vi "Low-Level Read.vi"(8 "error in (no error)":errorcluster, 9 "timeout ms (5000)":i32=5000, 11 "WebSockets in":refnum<class "WebSocket.lvclass">) -> (0 "error out":errorcluster, 1 "Opcode":T1=1 items=["Cont. Frame"=0, "Text"=1, "Binary"=2, "Ping"=9, "Pong"=10], 2 "Data":string, 3 "WebSockets out":refnum<class "WebSocket.lvclass">, 4 "Finished?":bool)   [LabVIEW 2013, in "WebSockets.lvlib" / "WebSocket.lvclass"]
doc: "Reads and decodes an incoming WebSockets message.\n\nOpcode: Opcode for the message.\nData: Contains the WebSockets payload\nFinished?: Determines whether the message is complete for fragmented messages. If false, must continue to read messages (continuation frames with opcode = 0) until Finished? is true."
uses:
  WebSocket.lvclass
  Opcodes.ctl
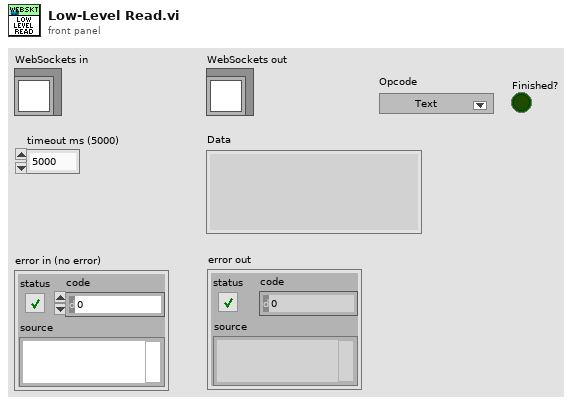
[diagram p1: front panel]
types:
  T1 = typedef "WebSockets.lvlib/WebSocket.lvclass/Opcodes.ctl" = u8
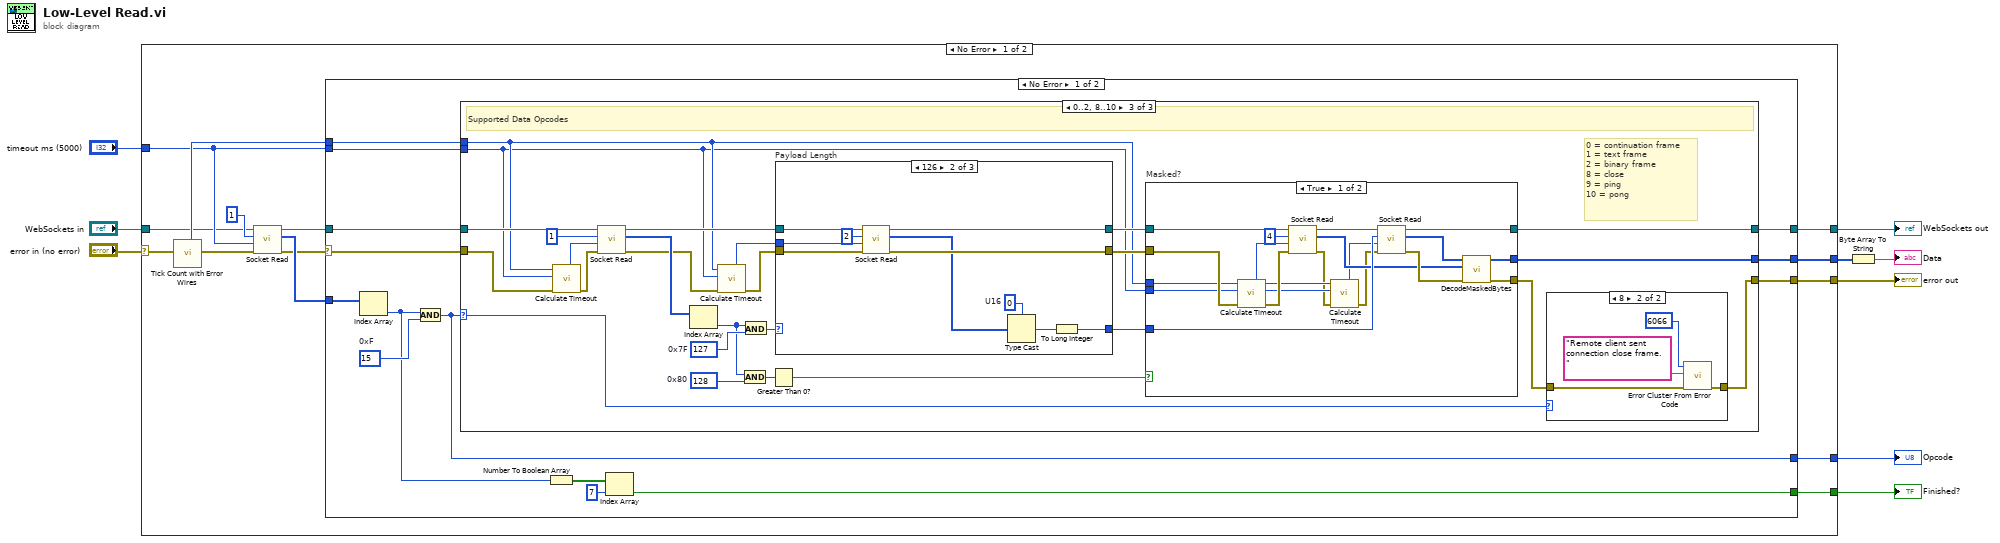
[diagram p0: block diagram]
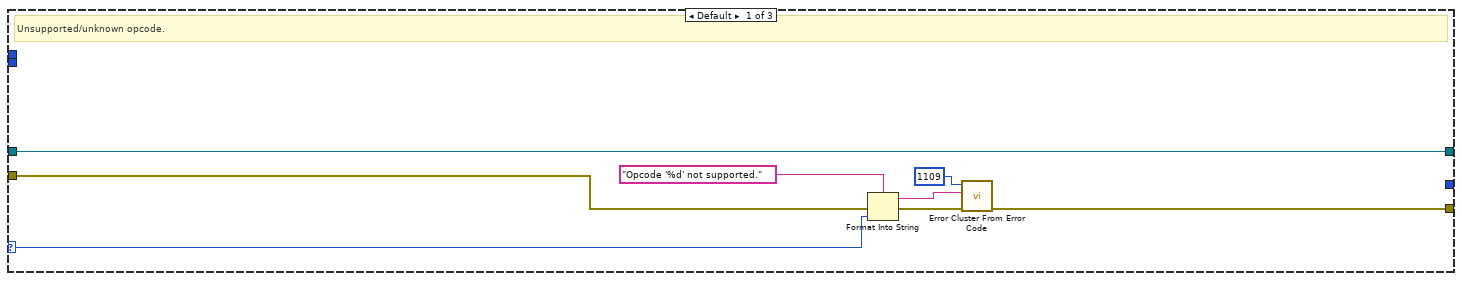
[diagram p2: hidden frame]
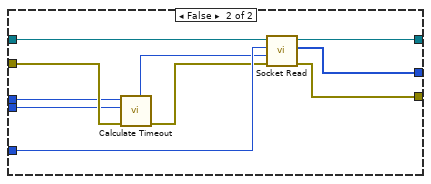
[diagram p5: hidden frame]
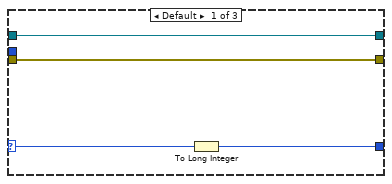
[diagram p6: hidden frame]
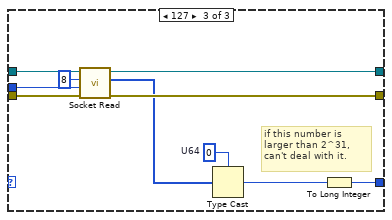
[diagram p7: hidden frame]
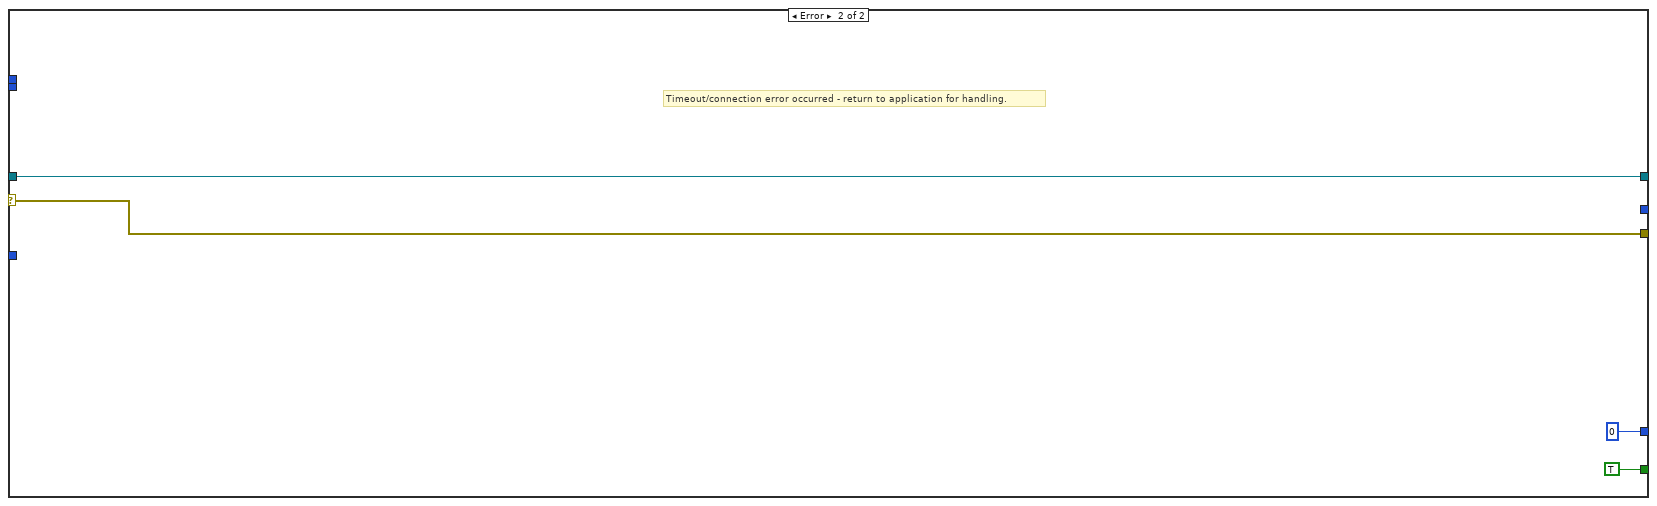
[diagram p8: hidden frame]
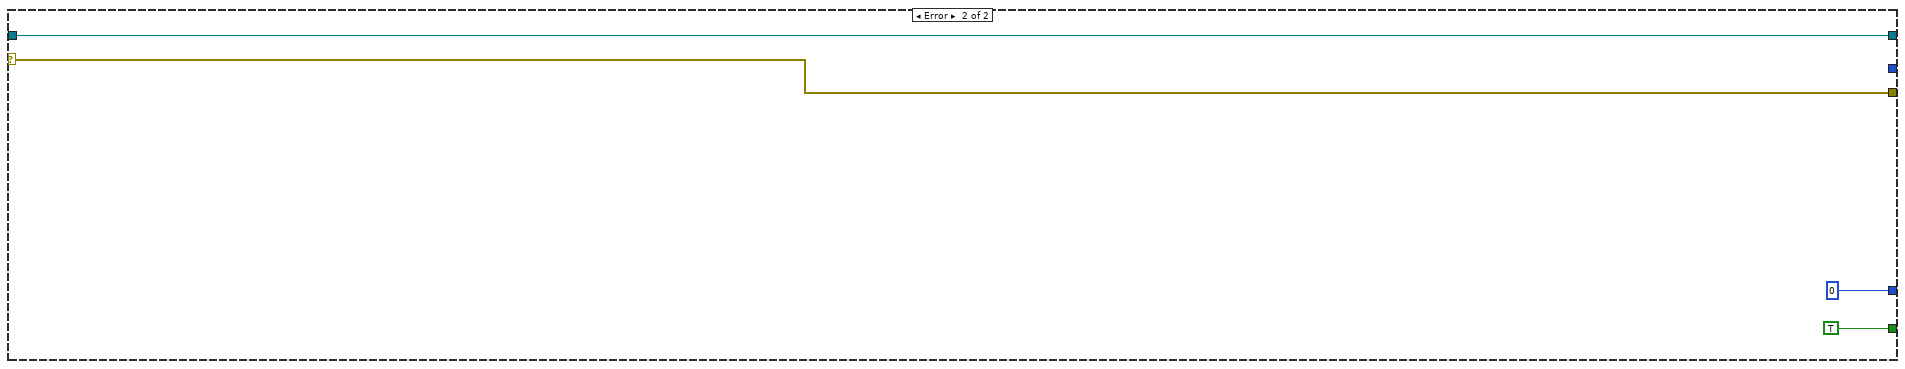
[diagram p9: hidden frame]
diagram:
  n1 = case shown="No Error" "error in (no error)" {
    selector: "error in (no error)" -> [w19 w138]
    tunnel: [w23 _] -> w9
    tunnel: [w22 w138] -> w7
    tunnel: "timeout ms (5000)" -> [w15 _]
    tunnel: [w21 u8 0] -> w4
    tunnel: [w20 TRUE] -> w5
    tunnel: "WebSockets in" -> [w11 w135]
    tunnel: [w10 w135] -> w1
    frame No Error {
      n2 = call "Tick Count with Error Wires.vi"("error in (no error)"=w19) -> ("error out"=w17:errorcluster, "millisecond timer value"=w18:u32)  [unwired: 9 in]
      n3 = call "Socket Read.vi"("error in (no error)"=w17, "timeout ms (5000)"=w15, "# bytes to read"=1 ("bytes to read"), "WebSocket in"=w11) -> ("error out"=w13:errorcluster, "Read Bytes"=w14:u8[], "WebSocket out"=w12:refnum<class "WebSocket.lvclass">)  [unwired: 5 in]
      n4 = case shown="No Error" w13 {
        selector: w13 -> [w33 w133]
        tunnel: w14 -> [w25 _]
        tunnel: w12 -> [w37 w134]
        tunnel: [w36 w134] -> w10
        tunnel: [w35 _] -> w23
        tunnel: [w34 w133] -> w22
        tunnel: [w31 u8 0] -> w21
        tunnel: [w28 TRUE] -> w20
        tunnel: w15 -> [w27 _]
        tunnel: w18 -> [w24 _]
        frame No Error {
          w32 = u8 15  # 0xF
          n5 = Index Array(array=w25) -> (element=w30:u8)  [unwired: 1 in]
          n6 = And(x=w30, y=w32) -> (x .and. y?=w31:u8)
          n7 = case shown="0..2, 8..10" w31 {
            selector: w31 -> [w39 _ w60]
            tunnel: w37 -> [w45 w46 w66]
            tunnel: [w45 w46 w73] -> w36
            tunnel: [_ _ w67] -> w35
            tunnel: [w44 w47 w58] -> w34
            tunnel: w33 -> [w43 w47 w55]
            tunnel: w27 -> [_ _ w48]
            tunnel: w24 -> [_ _ w49]
            frame Default {
              # "Unsupported/unknown opcode."
              n8 = Format Into String(format string="Opcode '%d' not supported.", error in=w43, w39) -> (resulting string=w41:string, error out=w42:errorcluster)  [unwired: 1 in]
              n9 = call <vilib>:"Error Cluster From Error Code.vi"("error in (no error)"=w42, "error message (\"\")"=w41, "error code (0)"=1109) -> ("error out"=w44:errorcluster)  [unwired: 6 in]
            }
            frame 3..7, 11..15 {
              # "3-7: Reserved non-control frames\n11-15: Reserved control frames"
              # "Reserved opcodes"
            }
            frame 0..2, 8..10 {
              w63 = u8 128  # 0x80
              w72 = u8 127  # 0x7F
              # "0 = continuation frame\n1 = text frame\n2 = binary frame\n8 = close\n9 = ping\n10 = pong"
              # "Supported Data Opcodes"
              n10 = call "Calculate Timeout.vi"("error in (no error)"=w55, "timeout ms"=w48, "t0"=w49) -> ("error out"=w54:errorcluster, "new timeout ms"=w52:i32)  [unwired: 6 in, 1 out]
              n11 = call "Socket Read.vi"("error in (no error)"=w54, "timeout ms (5000)"=w52, "# bytes to read"=1 ("bytes to read"), "WebSocket in"=w66) -> ("error out"=w53:errorcluster, "Read Bytes"=w57:u8[], "WebSocket out"=w65:refnum<class "WebSocket.lvclass">)  [unwired: 5 in]
              n12 = Index Array(array=w57) -> (element=w56:u8)  [unwired: 1 in]
              n13 = call "Calculate Timeout.vi"("error in (no error)"=w53, "timeout ms"=w48, "t0"=w49) -> ("error out"=w51:errorcluster, "new timeout ms"=w50:i32)  [unwired: 6 in, 1 out]
              n14 = And(x=w56, y=w63) -> (x .and. y?=w62:u8)
              n15 = And(x=w56, y=w72) -> (x .and. y?=w71:u8)
              n16 = Greater Than 0?(x=w62) -> (x > 0?=w61:bool)
              n17 = case "Payload Length" shown="126" w71 {
                selector: w71 -> [w109 _ _]
                tunnel: w65 -> [w110 w120 w129]
                tunnel: [w110 w119 w128] -> w70
                tunnel: [w108 w114 w127] -> w68
                tunnel: [w107 w117 w126] -> w69
                tunnel: w51 -> [w107 w116 w125]
                tunnel: w50 -> [_ w111 w121]
                frame Default {
                  n18 = To Long Integer(number=w109) -> (32bit integer=w108:i32)
                }
                frame 126 {
                  w113 = u16 0  # U16
                  n19 = call "Socket Read.vi"("error in (no error)"=w116, "timeout ms (5000)"=w111, "# bytes to read"=2 ("bytes to read"), "WebSocket in"=w120) -> ("error out"=w117:errorcluster, "Read Bytes"=w115:u8[], "WebSocket out"=w119:refnum<class "WebSocket.lvclass">)  [unwired: 5 in]
                  n20 = Type Cast(type=w113, x=w115) -> (*(type *) &x=w112:u16)
                  n21 = To Long Integer(number=w112) -> (32bit integer=w114:i32)
                }
                frame 127 {
                  w124 = u64 0  # U64
                  # "if this number is larger than 2^31, can't deal with it."
                  n22 = call "Socket Read.vi"("error in (no error)"=w125, "timeout ms (5000)"=w121, "# bytes to read"=8 ("bytes to read"), "WebSocket in"=w129) -> ("error out"=w126:errorcluster, "Read Bytes"=w122:u8[], "WebSocket out"=w128:refnum<class "WebSocket.lvclass">)  [unwired: 5 in]
                  n23 = Type Cast(type=w124, x=w122) -> (*(type *) &x=w123:u64)
                  n24 = To Long Integer(number=w123) -> (32bit integer=w127:i32)
                }
              }
              n25 = case "Masked?" shown="True" w61 {
                tunnel: [w96 w106] -> w73
                tunnel: w70 -> [w95 w105]
                tunnel: w69 -> [w86 w101]
                tunnel: w68 -> [w92 w104]
                tunnel: [w90 w102] -> w67
                tunnel: [w88 w103] -> w59
                tunnel: w49 -> [w83 w98]
                tunnel: w48 -> [w82 w97]
                frame True {
                  n26 = call "Calculate Timeout.vi"("error in (no error)"=w86, "timeout ms"=w82, "t0"=w83) -> ("error out"=w85:errorcluster, "new timeout ms"=w84:i32)  [unwired: 6 in, 1 out]
                  n27 = call "Socket Read.vi"("error in (no error)"=w85, "timeout ms (5000)"=w84, "# bytes to read"=4 ("bytes to read"), "WebSocket in"=w95) -> ("error out"=w81:errorcluster, "Read Bytes"=w87:u8[], "WebSocket out"=w94:refnum<class "WebSocket.lvclass">)  [unwired: 5 in]
                  n28 = call "Calculate Timeout.vi"("error in (no error)"=w81, "timeout ms"=w82, "t0"=w83) -> ("error out"=w80:errorcluster, "new timeout ms"=w79:i32)  [unwired: 6 in, 1 out]
                  n29 = call "Socket Read.vi"("error in (no error)"=w80, "timeout ms (5000)"=w79, "# bytes to read"=w92, "WebSocket in"=w94) -> ("error out"=w89:errorcluster, "Read Bytes"=w91:u8[], "WebSocket out"=w96:refnum<class "WebSocket.lvclass">)  [unwired: 5 in]
                  n30 = call "DecodeMaskedBytes.vi"("error in (no error)"=w89, "Mask Bytes"=w87, "Encoded Data"=w91) -> ("error out"=w88:errorcluster, "Decoded Data"=w90:u8[])  [unwired: 7 in]
                }
                frame False {
                  n31 = call "Calculate Timeout.vi"("error in (no error)"=w101, "timeout ms"=w97, "t0"=w98) -> ("error out"=w99:errorcluster, "new timeout ms"=w100:i32)  [unwired: 6 in, 1 out]
                  n32 = call "Socket Read.vi"("error in (no error)"=w99, "timeout ms (5000)"=w100, "# bytes to read"=w104, "WebSocket in"=w105) -> ("error out"=w103:errorcluster, "Read Bytes"=w102:u8[], "WebSocket out"=w106:refnum<class "WebSocket.lvclass">)  [unwired: 5 in]
                }
              }
              n33 = case shown="8" w60 {
                tunnel: w59 -> [w74 w76]
                tunnel: [w74 w75] -> w58
                frame Default {
                }
                frame 8 {
                  n34 = call <vilib>:"Error Cluster From Error Code.vi"("error in (no error)"=w76, "error message (\"\")"="Remote client sent connection close frame." ("error message (\"\")"), "error code (0)"=6066) -> ("error out"=w75:errorcluster)  [unwired: 6 in]
                }
              }
            }
          }
          n35 = Number To Boolean Array(number=w30) -> (Boolean array=w29:bool[])
          n36 = Index Array(array=w29, index=7) -> (element=w28:bool)
        }
        frame Error {
          # "Timeout/connection error occurred - return to application for handling."
        }
      }
    }
    frame Error {
    }
  }
  "error out" <- w7
  "Finished?" <- w5
  "Opcode" <- w4
  "WebSockets out" <- w1
  n37 = Byte Array To String(unsigned byte array=w9) -> (string=→"Data":string)
